vi "TCP Data Stream (old).vi"(0 "Address":string="localhost", 1 "Port":u16=2055 min=1025 step=1, 2 "Data IN":dbl[][](array[numeric]), 5 "Error IN":errorcluster, 6 "Mode":T1) -> (14 "Data OUT":dbl[][](array[numeric]), 15 "New Data?":bool, 16 "Connected?":bool, 19 "Error OUT":errorcluster)   [LabVIEW 2013]
uses:
  Type Defs/TCP Data Stream Mode.ctl
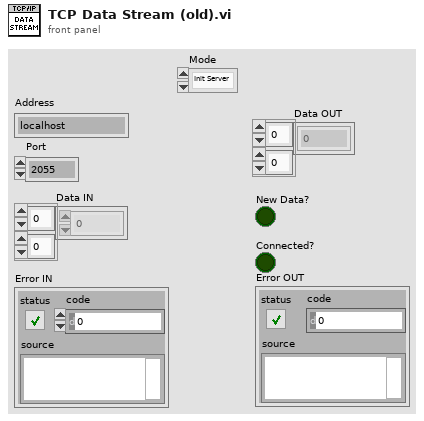
[diagram p1: front panel]
types:
  T1 = typedef "TCP Data Stream Mode.ctl" = enum16{"Init Server", "Init Client", "Write Data", "Read Data", "Close"}
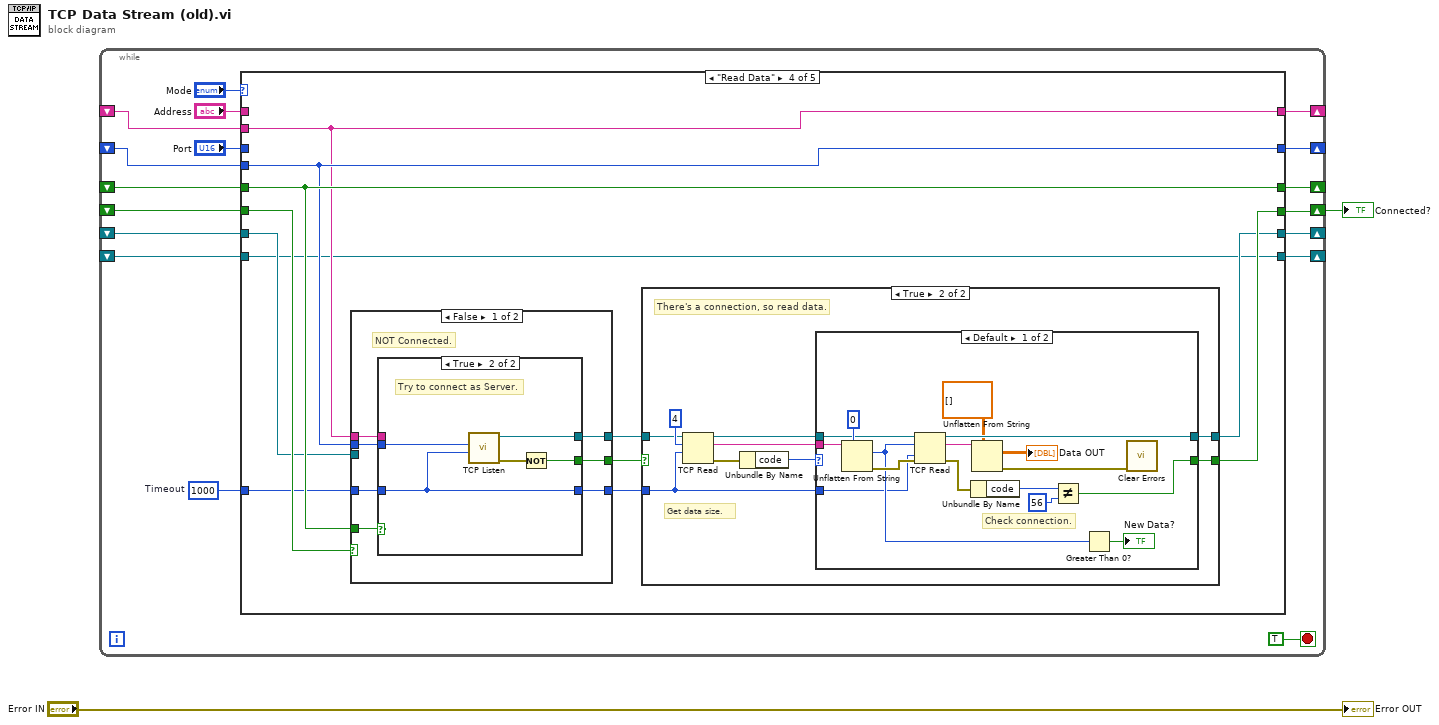
[diagram p0: block diagram]
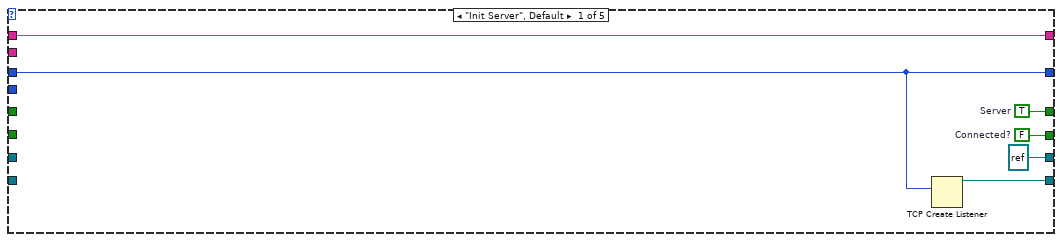
[diagram p2: hidden frame]
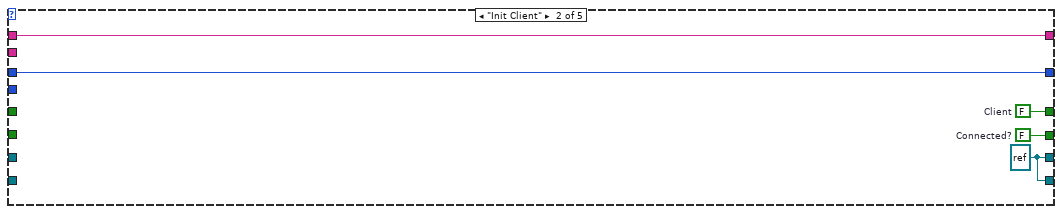
[diagram p3: hidden frame]
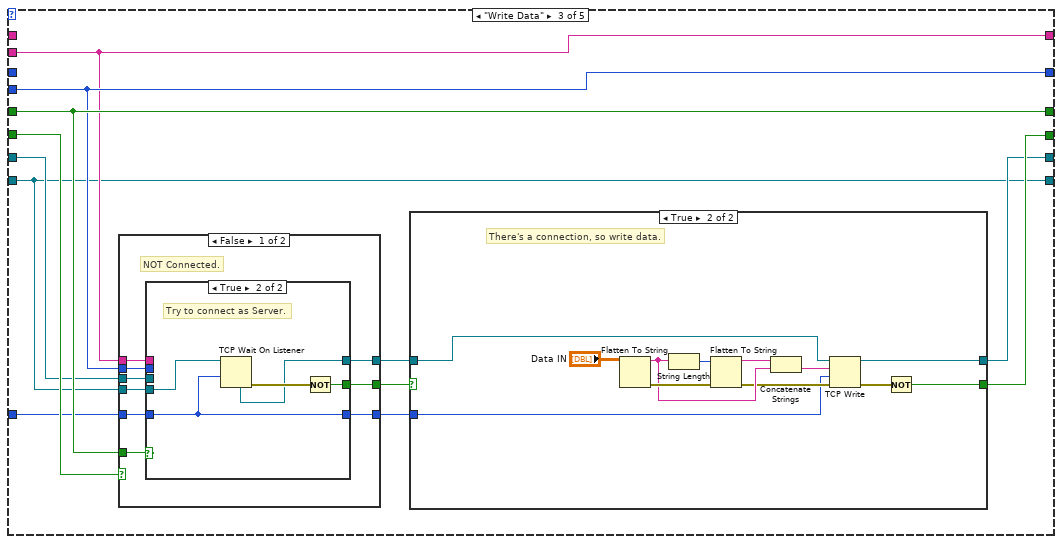
[diagram p4: hidden frame]
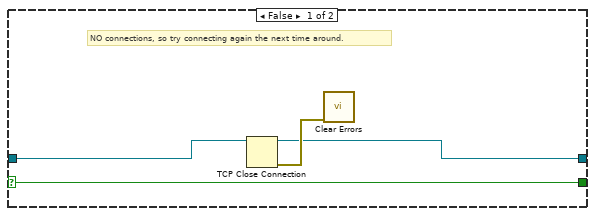
[diagram p5: hidden frame]
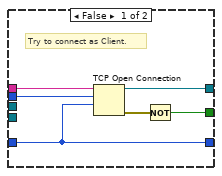
[diagram p6: hidden frame]
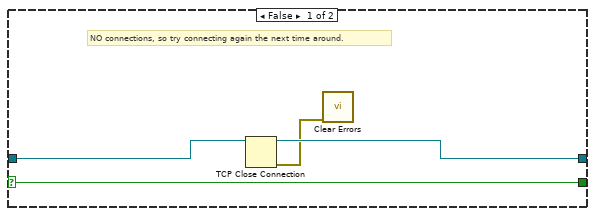
[diagram p8: hidden frame]
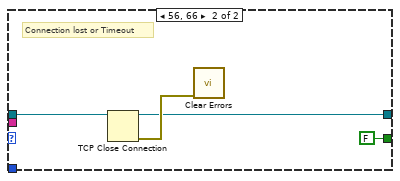
[diagram p9: hidden frame]
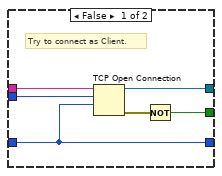
[diagram p10: hidden frame]
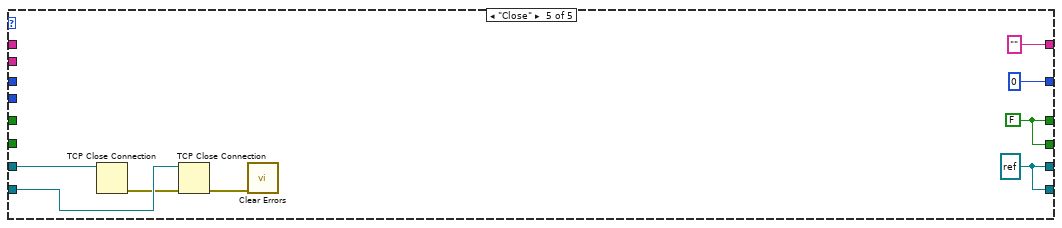
[diagram p12: hidden frame]
diagram:
  n1 = while {
    shift-right: [w16] -> _
    shift-left: _ -> [w9]
    shift-right: [w14] -> _
    shift-left: _ -> [w8]
    shift-right: [w13] -> _
    shift-left: _ -> [w12]
    shift-right: [w11] -> w2
    shift-left: _ -> [w10]
    shift-right: [w7] -> _
    shift-left: _ -> [w6]
    shift-right: [w4] -> _
    shift-left: _ -> [w3]
    stop <- TRUE stop-if-true
    w5 = 1000  # Timeout
    n2 = case shown="\"Read Data\"" "Mode" {
      tunnel: [w25 w30 w39 w90 "" ("Address")] -> w16
      tunnel: "Address" -> [w25 w30 _ _ _]
      tunnel: [w22 w29 w40 w91 u16 0 ("Port")] -> w14
      tunnel: "Port" -> [w22 w29 _ _ _]
      tunnel: [w24 w28 w41 w92 w153] -> w13
      tunnel: w12 -> [_ _ w41 w92 _]
      tunnel: [w23 w27 w37 w88 w153] -> w11
      tunnel: w10 -> [_ _ w42 w93 _]
      tunnel: w9 -> [_ _ w39 w90 _]
      tunnel: w8 -> [_ _ w40 w91 _]
      tunnel: [refnum<k5> refnum ("connection ID") w26 w35 w86 w152] -> w7
      tunnel: w6 -> [_ _ w34 w85 w151]
      tunnel: w5 -> [_ _ w33 w84 _]
      tunnel: [w20 w26 w31 w82 w152] -> w4
      tunnel: w3 -> [_ _ w31 w82 w150]
      frame "Init Server", Default {
        w23 = FALSE  # Connected?
        w24 = TRUE  # Server
        n3 = TCP Create Listener(10:w22) -> (3:w20:refnum<k5>)  [unwired: 4 in, 2 out]
      }
      frame "Init Client" {
        w26 = refnum<k5> refnum ("connection ID")
        w27 = FALSE  # Connected?
        w28 = FALSE  # Client
      }
      frame "Write Data" {
        n4 = case shown="False" w42 {
          selector: w42 -> [_ w81]
          tunnel: w41 -> [w67 _]
          tunnel: w40 -> [w66 _]
          tunnel: [w65 w80] -> w36
          tunnel: [w64 w81] -> w38
          tunnel: w39 -> [w63 _]
          tunnel: w34 -> [w60 w80]
          tunnel: w33 -> [w62 w79]
          tunnel: [w61 w79] -> w32
          tunnel: w31 -> [w59 _]
          frame False {
            # "NOT Connected."
            n5 = case shown="True" w67 {
              tunnel: w66 -> [w73 _]
              tunnel: [w72 w74] -> w65
              tunnel: [w69 w77] -> w64
              tunnel: w63 -> [w71 _]
              tunnel: w62 -> [w68 w78]
              tunnel: [w68 w78] -> w61
              tunnel: w60 -> [_ _]
              tunnel: w59 -> [_ w75]
              frame False {
                # "Try to connect as Client."
                n6 = TCP Open Connection(address=w71, remote port or service name=w73, timeout ms (60000)=w68) -> (connection ID=w72:refnum<k5>, error out=w70:errorcluster)  [unwired: 2 in]
                n7 = Not(x=w70) -> (.not. x?=w69:bool)
              }
              frame True {
                # "Try to connect as Server."
                n8 = TCP Wait On Listener(9:w78, 11:w75) -> (0:w76:errorcluster, 4:w74:refnum<k5>)  [unwired: 2 in, 3 out]
                n9 = Not(x=w76) -> (.not. x?=w77:bool)
              }
            }
          }
          frame True {
            # "Connected."
          }
        }
        n10 = case shown="True" w38 {
          selector: w38 -> [w46 _]
          tunnel: [w46 w56] -> w37
          tunnel: w36 -> [w44 w50]
          tunnel: [w43 w58] -> w35
          tunnel: w32 -> [_ w47]
          frame False {
            # "NO connections, so try connecting again the next time around."
            n11 = TCP Close Connection(connection ID=w44) -> (connection ID out=w43:refnum<k5>, error out=w45:errorcluster)  [unwired: 2 in]
            n12 = call <vilib>:"Clear Errors.vi"("error in (no error)"=w45) -> ()  [unwired: 6 in, 1 out]
          }
          frame True {
            # "There's a connection, so write data."
            n13 = Flatten To String(anything="Data IN") -> (data string=w52:string, error out=w55:errorcluster)  [unwired: 1 in, 3 out]
            n14 = String Length(string=w52) -> (length=w53:i32)
            n15 = Flatten To String(anything=w53, error in (no error)=w55) -> (data string=w54:string, error out=w51:errorcluster)  [unwired: 3 out]
            n16 = Concatenate Strings(w54, w52) -> (w49:string)
            n17 = TCP Write(connection ID=w50, data in=w49, error in (no error)=w51, 9:w47) -> (connection ID out=w58:refnum<k5>, error out=w57:errorcluster)  [unwired: 1 out]
            n18 = Not(x=w57) -> (.not. x?=w56:bool)
          }
        }
      }
      frame "Read Data" {
        n19 = case shown="False" w93 {
          selector: w93 -> [_ w147]
          tunnel: w92 -> [w133 _]
          tunnel: w91 -> [w132 _]
          tunnel: [w131 w146] -> w87
          tunnel: [w130 w147] -> w89
          tunnel: w90 -> [w129 _]
          tunnel: w85 -> [_ w146]
          tunnel: w84 -> [w128 w145]
          tunnel: [w127 w145] -> w83
          frame False {
            # "NOT Connected."
            n20 = case shown="True" w133 {
              tunnel: w132 -> [w139 w144]
              tunnel: [w138 w143] -> w131
              tunnel: [w135 w141] -> w130
              tunnel: w129 -> [w137 _]
              tunnel: w128 -> [w134 w140]
              tunnel: [w134 w140] -> w127
              frame False {
                # "Try to connect as Client."
                n21 = TCP Open Connection(address=w137, remote port or service name=w139, timeout ms (60000)=w134) -> (connection ID=w138:refnum<k5>, error out=w136:errorcluster)  [unwired: 2 in]
                n22 = Not(x=w136) -> (.not. x?=w135:bool)
              }
              frame True {
                # "Try to connect as Server."
                n23 = call <vilib>:"TCP Listen.vi"("timeout ms (wait forever: -1)"=w140, "port"=w144) -> ("error out"=w142:errorcluster, "connection ID"=w143:refnum<k5>)  [unwired: 5 in, 3 out]
                n24 = Not(x=w142) -> (.not. x?=w141:bool)
              }
            }
          }
          frame True {
            # "Connected."
          }
        }
        n25 = case shown="True" w89 {
          selector: w89 -> [w97 _]
          tunnel: [w97 w104] -> w88
          tunnel: w87 -> [w96 w105]
          tunnel: [w95 w102] -> w86
          tunnel: w83 -> [_ w100]
          frame False {
            # "NO connections, so try connecting again the next time around."
            n26 = TCP Close Connection(connection ID=w96) -> (connection ID out=w95:refnum<k5>, error out=w94:errorcluster)  [unwired: 2 in]
            n27 = call <vilib>:"Clear Errors.vi"("error in (no error)"=w94) -> ()  [unwired: 6 in, 1 out]
          }
          frame True {
            # "Get data size."
            # "There's a connection, so read data."
            n28 = TCP Read(connection ID=w105, bytes to read=4, 9:w100) -> (connection ID out=w103:refnum<k5>, data out=w101:string, error out=w99:errorcluster)  [unwired: 1 in, 1 out]
            n29 = Unbundle By Name(w99) -> ("code"=w98:i32)
            n30 = case shown="Default" w98 {
              tunnel: [w115 FALSE] -> w104
              tunnel: [w113 w124] -> w102
              tunnel: w103 -> [w120 w126]
              tunnel: w101 -> [w119 _]
              tunnel: w100 -> [w107 _]
              frame Default {
                # "Check connection."
                n31 = Unflatten From String(type=0 ("bytes to read"), binary string=w119) -> (value=w110:i32, error out=w122:errorcluster)  [unwired: 2 in, 2 out]
                n32 = TCP Read(connection ID=w120, bytes to read=w110, error in (no error)=w122, 9:w107) -> (connection ID out=w113:refnum<k5>, data out=w114:string, error out=w116:errorcluster)  [unwired: 1 in]
                n33 = Unbundle By Name(w116) -> ("code"=w118:i32)
                n34 = Unflatten From String(type=dbl[][] [] ("Data OUT"), binary string=w114) -> (value=→"Data OUT":dbl[][], error out=w108:errorcluster)  [unwired: 1 in, 3 out]
                n35 = Not Equal?(x=w118, y=56) -> (x != y?=w115:bool)
                n36 = Greater Than 0?(x=w110) -> (x > 0?=→"New Data?":bool)
                n37 = call <vilib>:"Clear Errors.vi"("error in (no error)"=w108) -> ()  [unwired: 6 in, 1 out]
              }
              frame 56, 66 {
                # "Connection lost or Timeout"
                n38 = TCP Close Connection(connection ID=w126) -> (connection ID out=w124:refnum<k5>, error out=w125:errorcluster)  [unwired: 2 in]
                n39 = call <vilib>:"Clear Errors.vi"("error in (no error)"=w125) -> ()  [unwired: 6 in, 1 out]
              }
            }
          }
        }
      }
      frame "Close" {
        w152 = refnum<k5> refnum ("connection ID")
        w153 = FALSE ("Client")
        n40 = TCP Close Connection(connection ID=w151) -> (error out=w149:errorcluster)  [unwired: 2 in, 1 out]
        n41 = TCP Close Connection(connection ID=w150, error in (no error)=w149) -> (error out=w148:errorcluster)  [unwired: 1 in, 1 out]
        n42 = call <vilib>:"Clear Errors.vi"("error in (no error)"=w148) -> ()  [unwired: 6 in, 1 out]
      }
    }
  }
  "Connected?" <- w2
  "Error OUT" <- "Error IN"
